vi "Create files.vi"(8 "error in (no error)":errorcluster, 11 "INI Refnum in":T1) -> (0 "error out":errorcluster, 3 "INI Refnum out":T1)   [LabVIEW 2015]
uses:
  <vilib>/Utility/config.llb/Config Data RefNum.ctl
  <vilib>/Utility/config.llb/Read Key (Path).vi
  <vilib>/Utility/config.llb/NI_LVConfig.lvlib
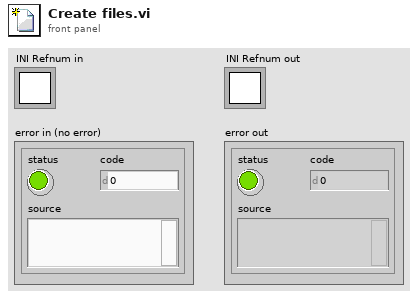
[diagram p1: front panel]
types:
  T1 = typedef "NI_LVConfig.lvlib/Config Data RefNum.ctl" = refnum<k1>
  T2 = enum16{"open", "replace", "create", "open or create", "replace or create", "replace or create with confirmation"}
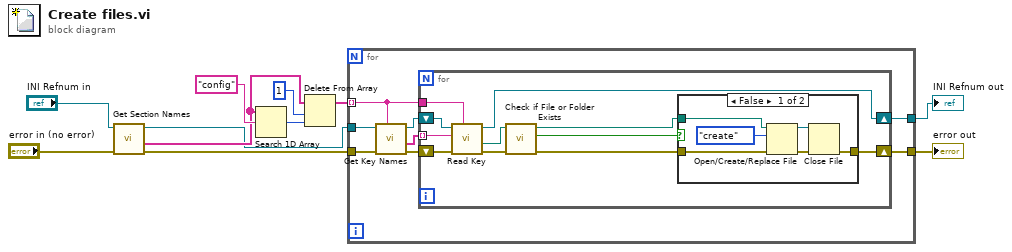
[diagram p0: block diagram]
diagram:
  n1 = call <vilib>:"Get Section Names.vi"("error in (no error)"="error in (no error)", "refnum"="INI Refnum in") -> ("error out"=w4:errorcluster, "section names"=w7:string[], "refnum out"=w3:T1)  [unwired: 7 in]
  n2 = Search 1D Array(1D array=w7, element="config") -> (index of element=w9:i32)  [unwired: 1 in]
  n3 = Delete From Array(array=w7, length=1, index=w9) -> (array with subset deleted=w11:string[])  [unwired: 1 out]
  n4 = for {
    tunnel: w3 -> [w19]
    tunnel: w4 -> [w18]
    tunnel: w11 -> [w15] mode=indexing
    tunnel: [w13] -> w6
    tunnel: [w12] -> w5
    n5 = call <vilib>:"Get Key Names.vi"("section"=w15, "error in (no error)"=w18, "refnum"=w19) -> ("error out"=w14:errorcluster, "key names"=w16:string[], "refnum out"=w17:T1)  [unwired: 5 in, 1 out]
    n6 = for {
      tunnel: w16 -> [w29] mode=indexing
      tunnel: w15 -> [w28]
      shift-right: [w21] -> w12
      shift-left: w17 -> [w30]
      shift-right: [w22] -> w13
      shift-left: w14 -> [w25]
      n7 = call-poly <vilib>:"Read Key.vi"("section"=w28, "error in (no error)"=w25, "key"=w29, "refnum"=w30) -> ("error out"=w26:errorcluster, "value"=w27:path, "refnum out"=w21:T1)  [unwired: 4 in, 1 out]
      n8 = call <vilib>:"Check if File or Folder Exists.vi"("error in (no error)"=w26, "path"=w27) -> ("error out"=w23:errorcluster, "file or folder exists?"=w24:bool, "dup path"=w20:path)  [unwired: 7 in]
      n9 = case shown="False" w24 {
        tunnel: w20 -> [w36 _]
        tunnel: w23 -> [w35 w37]
        tunnel: [w31 w37] -> w22
        frame False {
          n10 = Open/Create/Replace File(file path (use dialog)=w36, error in=w35, operation (0:open)=T2."create") -> (refnum out=w32:refnum<file>, error out=w33:errorcluster)  [unwired: 3 in, 1 out]
          n11 = Close File(refnum=w32, error in=w33) -> (error out=w31:errorcluster)  [unwired: 1 out]
        }
        frame True {
        }
      }
    }
  }
  "error out" <- w6
  "INI Refnum out" <- w5
